vi "line_profile(SubVI).vi"(8 "error in":errorcluster, 11 "image src":T1) -> (0 "error out":errorcluster, 2 "image Out":T1, 3 "Line Graph":cluster{"x0":sgl, "dx":sgl, "Pixels Line":sgl[]} {"Pixels Line" format="%.2f"; "dx" format="%.2f"; "x0" format="%.2f"})   [LabVIEW 2020]
doc: "Permette di visualizzare i livelli di grigio di pixel che si trovano su una linea che si può disegnare sull'immagine in ingresso (Image SRC). Richiede in ingresso un'immagine in bianco e nero. Fornisce in uscita l'immagine e il grafico dei livelli di grigio del pixel."
uses:
  <vilib>/vision/Image Controls.llb/IMAQ Image.ctl
  <vilib>/vision/NI_Vision_Development_Module.lvlib
panel:
  out "Array":dbl[](array[numeric])
  out "Waveform Graph":cluster{"x0":sgl, "dx":sgl, "Pixels Line":sgl[]}(graph)
  in  "stop":bool
  out "grey scale image":T1(plugin-control)
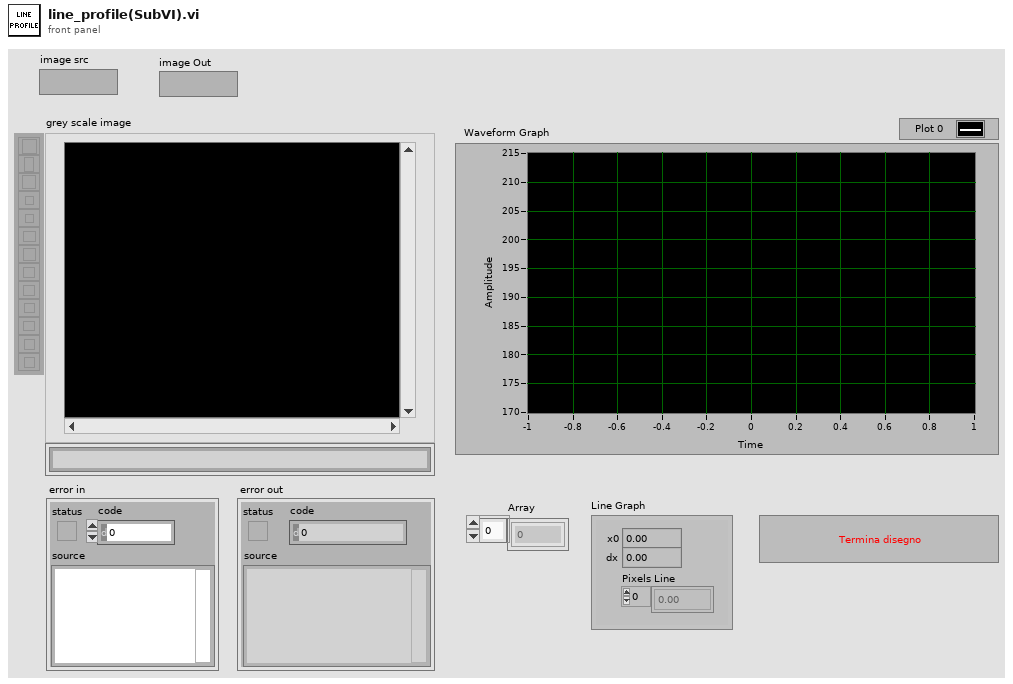
[diagram p1: front panel]
types:
  T1 = typedef "IMAQ Image.ctl" = refnum<image>
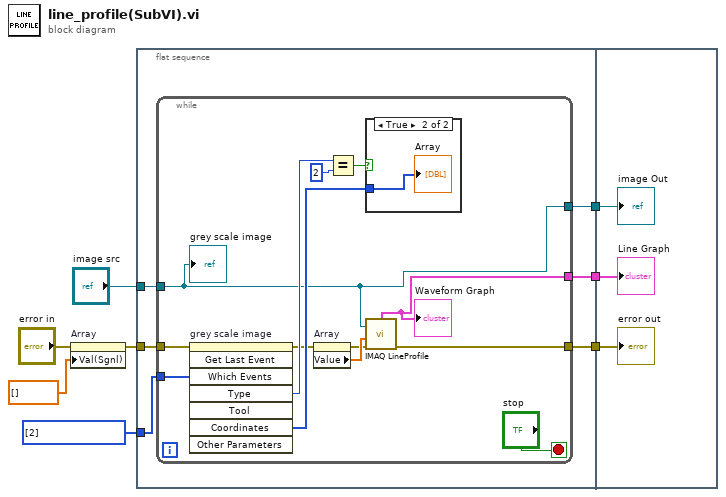
[diagram p0: block diagram]
diagram:
  w6 = i32[] [2] items=["No Event"=0, "Click Event"=1, "Draw Event"=2, "Size Event"=4, "Scroll Event"=5, "Double Click Event"=8] ("Which Events")
  n1 = property on="Array" class="Arr (strict)"(error in="error in", "Val(Sgnl)"=dbl[] [] ("Value (Signaling)")) -> (error out=w4:errorcluster)  [unwired: 1 in, 1 out]
  n2 = flat-sequence {
    tunnel: w6 -> [w14]
    tunnel: "image src" -> [w13]
    tunnel: w4 -> [w12]
    tunnel: [w11] -> w3
    tunnel: [w10] -> w2
    tunnel: [w9] -> w1
    tunnel: w3 -> [w31]
    tunnel: w2 -> [w30]
    tunnel: w1 -> [w29]
    frame #0 {
      n3 = while {
        tunnel: [w22] -> w11
        tunnel: w14 -> [w26]
        tunnel: w13 -> [w15]
        tunnel: w12 -> [w18]
        tunnel: [w16] -> w10
        tunnel: [w15] -> w9
        stop <- "stop" stop-if-true
        n4 = invoke on="grey scale image" class="ImageControl" method="Get Last Event"(error in=w18, "Which Events"=w26) -> (error out=w17:errorcluster, "Type"=w25:i32, "Coordinates"=w21:i32[])  [unwired: 6 in, 5 out]
        n5 = property on="Array" class="Arr (strict)"(error in=w17) -> (error out=w19:errorcluster, "Value"=w20:dbl[])  [unwired: 1 in, 1 out]
        n6 = Equal?(x=w25, y=2) -> (x = y?=w23:bool)
        n7 = case shown="True" w23 {
          tunnel: w21 -> [_ w28]
          frame False {
          }
          frame True {
            "Array" <- w28
          }
        }
        n8 = call "IMAQ LineProfile"("error in (no error)"=w19, "Line Coordinates"=w20, "Image"=w15) -> ("error out"=w22:errorcluster, "Line Graph"=w16:cluster{"x0":sgl, "dx":sgl, "Pixels Line":sgl[]})  [unwired: 2 in, 2 out]
        "Waveform Graph" <- w16
        "grey scale image" <- w15
      }
    }
    frame #1 {
      "image Out" <- w29
      "Line Graph" <- w30
      "error out" <- w31
    }
  }
